vi "Subscribe to Data Broadcast.vi"(7 "Message Priority (Normal)":T1=enum."Normal", 8 "error in (no error)":errorcluster, 9 "Concrete Data Msg":refnum<class "Data Msg.lvclass">, 10 "Listener NQR":refnum<class "Message Enqueuer.lvclass">, 11 "Subscription Token In":refnum<class "Subscription Token.lvclass">) -> (0 "error out":errorcluster, 3 "Subscription Token Out":refnum<class "Subscription Token.lvclass">)   [LabVIEW 2016, in "Data Broadcasting.lvlib" / "Subscription Token.lvclass"]
doc: "Subscribes a Listener to a data broadcast so that it will receive the next broadcast update. Listeners are identified by their <b>NQR</b> (Enqueuer). Each Listener is sent its own <b>Concrete Data Msg</b>.\n\n\n-------------\nCopyright (c) 2013, Staab Engineering, a Texas Limited Liability Company\nAll rights reserved.\n\nRedistribution and use in source and binary forms, with or without modification, are permitted provided that the following conditions are met:\n\n1. Redistributions of source code must retain the above copyright notice, this list of conditions and the following disclaimer.\n2. Redistributions in binary form must reproduce the above copyright notice, this list of conditions and the following disclaimer in the documentation and/or other materials provided with the distribution.\n\nTHIS SOFTWARE IS PROVIDED BY THE COPYRIGHT HOLDERS AND CONTRIBUTORS \"AS IS\" AND ANY EXPRESS OR IMPLIED WARRANTIES, INCLUDING, BUT NOT LIMITED TO, THE IMPLIED WARRANTIES OF MERCHANTABILITY AND FITNESS FOR A PARTICULAR PURPOSE ARE DISCLAIMED. IN NO EVENT SHALL THE COPYRIGHT HOLDER OR CONTRIBUTORS BE LIABLE FOR ANY DIRECT, INDIRECT, INCIDENTAL, SPECIAL, EXEMPLARY, OR CONSEQUENTIAL DAMAGES (INCLUDING, BUT NOT LIMITED TO, PROCUREMENT OF SUBSTITUTE GOODS OR SERVICES; LOSS OF USE, DATA, OR PROFITS; OR BUSINESS INTERRUPTION) HOWEVER CAUSED AND ON ANY THEORY OF LIABILITY, WHETHER IN CONTRACT, STRICT LIABILITY, OR TORT (INCLUDING NEGLIGENCE OR OTHERWISE) ARISING IN ANY WAY OUT OF THE USE OF THIS SOFTWARE, EVEN IF ADVISED OF THE POSSIBILITY OF SUCH DAMAGE."
uses:
  <userlib>/_Frameworks/Staab/AF Data Broadcasting/Data Broadcasting/Subscription Token/Subscription Token.lvclass
  <vilib>/ActorFramework/Message Enqueuer/Message Enqueuer.lvclass
  <vilib>/ActorFramework/Message Enqueuer/Message Priority.ctl
  <userlib>/_Frameworks/Staab/AF Data Broadcasting/Data Broadcasting/Data Msg/Data Msg.lvclass
  <userlib>/_Frameworks/Staab/AF Data Broadcasting/Data Broadcasting/Subscription Token/Subscription Token.lvclass/Subscription Token.ctl
  <vilib>/ActorFramework/Message Enqueuer/Message Enqueuer.lvclass/Message Enqueuer.ctl
  <userlib>/_Frameworks/Staab/AF Data Broadcasting/Data Broadcasting/Registration Msg/Registration Msg.lvclass
  C:/Program Files (x86)/National Instruments/LabVIEW 2016/vi.lib/ActorFramework/Message/Message.lvclass
  <vilib>/ActorFramework/Message Priority Queue/Priority Enqueue.vi
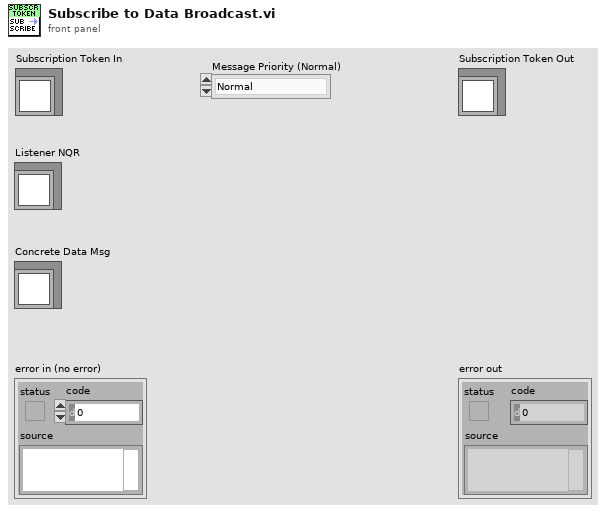
[diagram p1: front panel]
types:
  T1 = typedef "Actor Framework.lvlib/Message Enqueuer.lvclass/Message Priority.ctl" = enum16{"Low", "Normal", "High"}
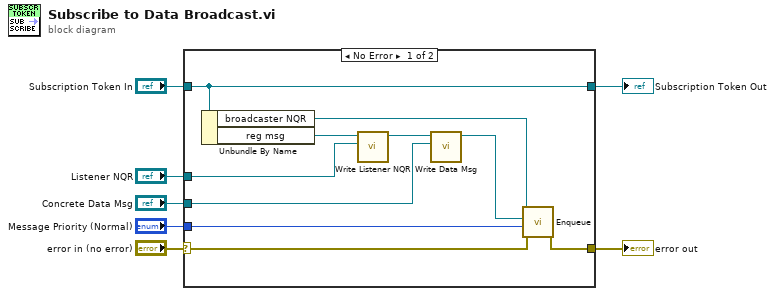
[diagram p0: block diagram]
diagram:
  n1 = case shown="No Error" "error in (no error)" {
    selector: "error in (no error)" -> [w17 w19]
    tunnel: [w16 w19] -> w6
    tunnel: "Subscription Token In" -> [w8 w18]
    tunnel: "Message Priority (Normal)" -> [w14 _]
    tunnel: "Listener NQR" -> [w11 _]
    tunnel: "Concrete Data Msg" -> [w9 _]
    tunnel: [w8 w18] -> w1
    frame No Error {
      n2 = Unbundle By Name(w8) -> ("broadcaster NQR"=w15:refnum<class "Message Enqueuer.lvclass">, "reg msg"=w12:refnum<class "Registration Msg.lvclass">)
      n3 = call <userlib>:"Write Listener NQR.vi"("Listener NQR"=w11, "Registration Msg In"=w12) -> ("Registration Msg Out"=w13:refnum<class "Registration Msg.lvclass">)  [unwired: 9 in]
      n4 = call <userlib>:"Write Data Msg.vi"("Data Msg"=w9, "Registration Msg In"=w13) -> ("Registration Msg Out"=w10:refnum<class "Registration Msg.lvclass">)  [unwired: 9 in]
      n5 = call <vilib>:"Enqueue.vi"("error in (no error)"=w17, "Message Priority (Normal)"=w14, "Message"=w10, "Message Enqueuer in"=w15) -> ("error out"=w16:errorcluster)  [unwired: 6 in, 1 out]
    }
    frame Error {
    }
  }
  "error out" <- w6
  "Subscription Token Out" <- w1
